vi "Unit Test.vi"() -> ()   [LabVIEW 2017]
uses:
  builds/Oven.lvlibp/Custom Controls/Message Type.ctl
  Custom Controls/Message Type.ctl
  builds/Oven.lvlibp/Oven.lvclass
  builds/Oven.lvlibp
  Oven.lvlib
panel:
  out "Oven Status":u32(colorbox)=1985280
  out "Over Temp":bool
  out "Current Temperature":dbl
  out "Elapsed Time":dbl
  out "Interlock":bool
  in  "Oven State:":bool
  in  "Temperature Setpoint":dbl
  in  "stop":bool
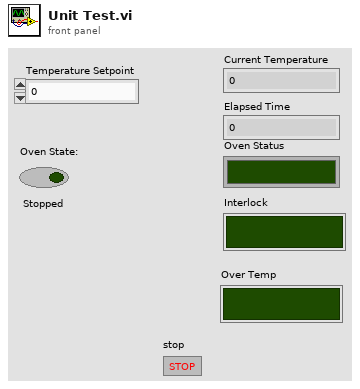
[diagram p1: front panel]
types:
  T1 = typedef "Oven.lvlibp/Message Type.ctl" = enum16{"Start", "Stop", "Set Temperature", "Get Temperature"}
  T2 = typedef "Oven.lvlib/Message Type.ctl" = enum16{"Start", "Stop", "Set Temperature", "Get Temperature"}
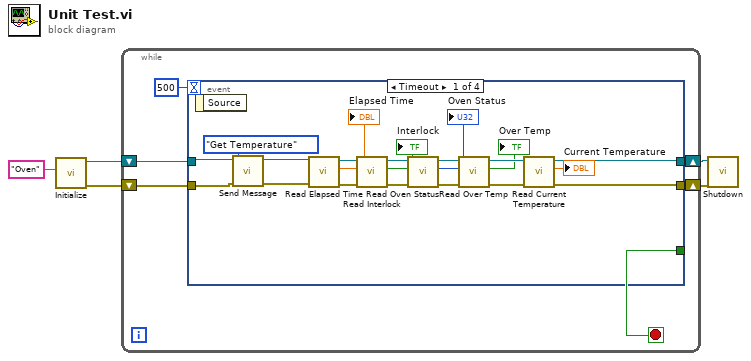
[diagram p0: block diagram]
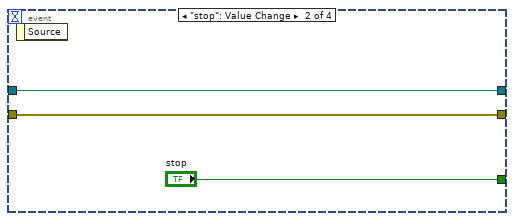
[diagram p2: hidden frame]
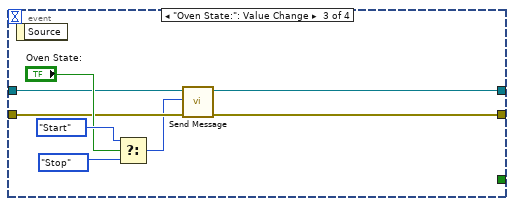
[diagram p3: hidden frame]
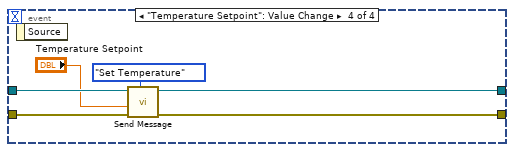
[diagram p4: hidden frame]
diagram:
  n1 = call "Initialize.vi"("Device"="Oven") -> ("error out"=w4:errorcluster, "Oven out"=w5:refnum<class "Oven.lvclass">)  [unwired: 9 in]
  n2 = while {
    shift-right: [w9] -> w2
    shift-left: w5 -> [w11]
    shift-right: [w8] -> w1
    shift-left: w4 -> [w10]
    stop <- w7 stop-if-true
    n3 = event shown="[0] Timeout" {
      selector: _ -> [_ _ _ _]
      dyn-events: _ -> [_ _ _ _]
      timeout: 500 -> [_ _ _ _]
      tunnel: w11 -> [w31 w34 w39 w48]
      tunnel: w10 -> [w30 w33 w36 w47]
      tunnel: [w18 w34 w38 w44] -> w9
      tunnel: [w17 w33 w37 w43] -> w8
      tunnel: [_ "stop" _ _] -> w7
      event Timeout {
        n4 = event-data() -> ()  [unwired: 1 in, 1 out]
        n5 = call-dynamic "Send Message.vi"("error in (no error)"=w30, "Message to Send"=Message_Type."Get Temperature", "Oven in"=w31) -> ("error out"=w28:errorcluster, "Oven out"=w27:refnum<class "Oven.lvclass">)  [unwired: 7 in]
        n6 = call "Read Elapsed Time.vi"("error in (no error)"=w28, "Oven in"=w27) -> ("error out"=w26:errorcluster, "Elapsed Time"=→"Elapsed Time":dbl, "Oven out"=w25:refnum<class "Oven.lvclass">)  [unwired: 7 in]
        n7 = call "Read Interlock.vi"("error in (no error)"=w26, "Oven in"=w25) -> ("error out"=w23:errorcluster, "Interlock"=→"Interlock":bool, "Oven out"=w24:refnum<class "Oven.lvclass">)  [unwired: 7 in]
        n8 = call "Read Oven Status.vi"("error in (no error)"=w23, "Oven in"=w24) -> ("error out"=w21:errorcluster, "Oven Status"=→"Oven Status":u32, "Oven out"=w22:refnum<class "Oven.lvclass">)  [unwired: 7 in]
        n9 = call "Read Over Temp.vi"("error in (no error)"=w21, "Oven in"=w22) -> ("error out"=w20:errorcluster, "Over Temp"=→"Over Temp":bool, "Oven out"=w19:refnum<class "Oven.lvclass">)  [unwired: 7 in]
        n10 = call "Read Current Temperature.vi"("error in (no error)"=w20, "Oven in"=w19) -> ("error out"=w17:errorcluster, "Current Temperature"=→"Current Temperature":dbl, "Oven out"=w18:refnum<class "Oven.lvclass">)  [unwired: 7 in]
      }
      event "stop": Value Change {
        n11 = event-data() -> ()  [unwired: 1 in, 1 out]
      }
      event "Oven State:": Value Change {
        n12 = event-data() -> ()  [unwired: 1 in, 1 out]
        n13 = Select(t=Message_Type."Start" ("Message to Send"), s="Oven State:", f=Message_Type."Stop" ("Message to Send")) -> (s? t:f=w35:T2)
        n14 = call-dynamic "Send Message.vi"("error in (no error)"=w36, "Message to Send"=w35, "Oven in"=w39) -> ("error out"=w37:errorcluster, "Oven out"=w38:refnum<class "Oven.lvclass">)  [unwired: 7 in]
      }
      event "Temperature Setpoint": Value Change {
        n15 = event-data() -> ()  [unwired: 1 in, 1 out]
        n16 = call-dynamic "Send Message.vi"("error in (no error)"=w47, "Value"="Temperature Setpoint", "Message to Send"=Message_Type."Set Temperature", "Oven in"=w48) -> ("error out"=w43:errorcluster, "Oven out"=w44:refnum<class "Oven.lvclass">)  [unwired: 6 in]
      }
    }
  }
  n17 = call "Shutdown.vi"("error in"=w1, "Oven in"=w2) -> ()  [unwired: 8 in, 2 out]
